vi "Laser.vi"() -> ()   [LabVIEW 2013]
doc: "Пограмма управления мишенью лазерного источника ионов."
uses:
  <vilib>/Utility/error.llb/DialogType.ctl
  <vilib>/Utility/inputDevices.llb/closeMouse.vi
  <vilib>/Utility/inputDevices.llb/mouseAcquire.vi
panel:
  in  "?":enum32{" Графики", " Настройки соединения"}(tab)
  out "Slide X axis":u8(slide) max=100 scale=0.0..100.0
  out "Slide Y axis":u8(slide) max=50 step=1
  in  "Коорд. y положение панели":u16
  in  "Коорд. X положение панели":u16
  in  "Add Button":bool
  in  "Коорд. Y":u16
  in  "Коорд. X":u16
  in  "размер, Y":dbl step=10.0
  in  "размер, X":dbl
  in  "Снимок":bool
  in  "Запись в файл":bool
  out "con err":bool caption="Connect"
  out "Con":bool
  out "warning1":string
  out "data out":string
  in  "thickness":u16 step=1
  out "Mouse on Pane pos Horizontal":i32
  out "Mouse on Pane pos Vertical":i32
  in  "in picture":picture
  in  "порт":u16=4001
  in  "IP-адрес":string="10.10.10.2"
  in  "Disconnect":bool caption="Disconn"
  out "Connected":bool
  in  "Connect":bool
  out "TCP error source":string
  in  "stop":bool
  out "read_error_indicator":bool
  in  "Connect 2":bool caption="Connect"
  in  "Компактный вид":bool
  out "resize Fl":bool caption="Disconn"
  in  "flag1":bool caption="Disconn"
  out "x+1":dbl
  out "connection ID":refnum<k5>
types:
  T1 = typedef "DialogType.ctl" = u16
  T2 = typedef "imagedata.ctl" = cluster{"image type":i32, "image depth":i32, "image":u8[], "mask":u8[], "colors":u32[], "Rectangle":cluster{"left":i16, "top":i16, "right":i16, "bottom":i16}}
  T3 = cluster{"Коорд. X положение панели":u16, "Коорд. y положение панели":u16}
  T4 = cluster{"Horizontal":i32, "Vertical":i32, "Scrolling":i32}
  T5 = typedef "LVRectTypeDef.ctl" = cluster{"Left":i16, "Top":i16, "Right":i16, "Bottom":i16}
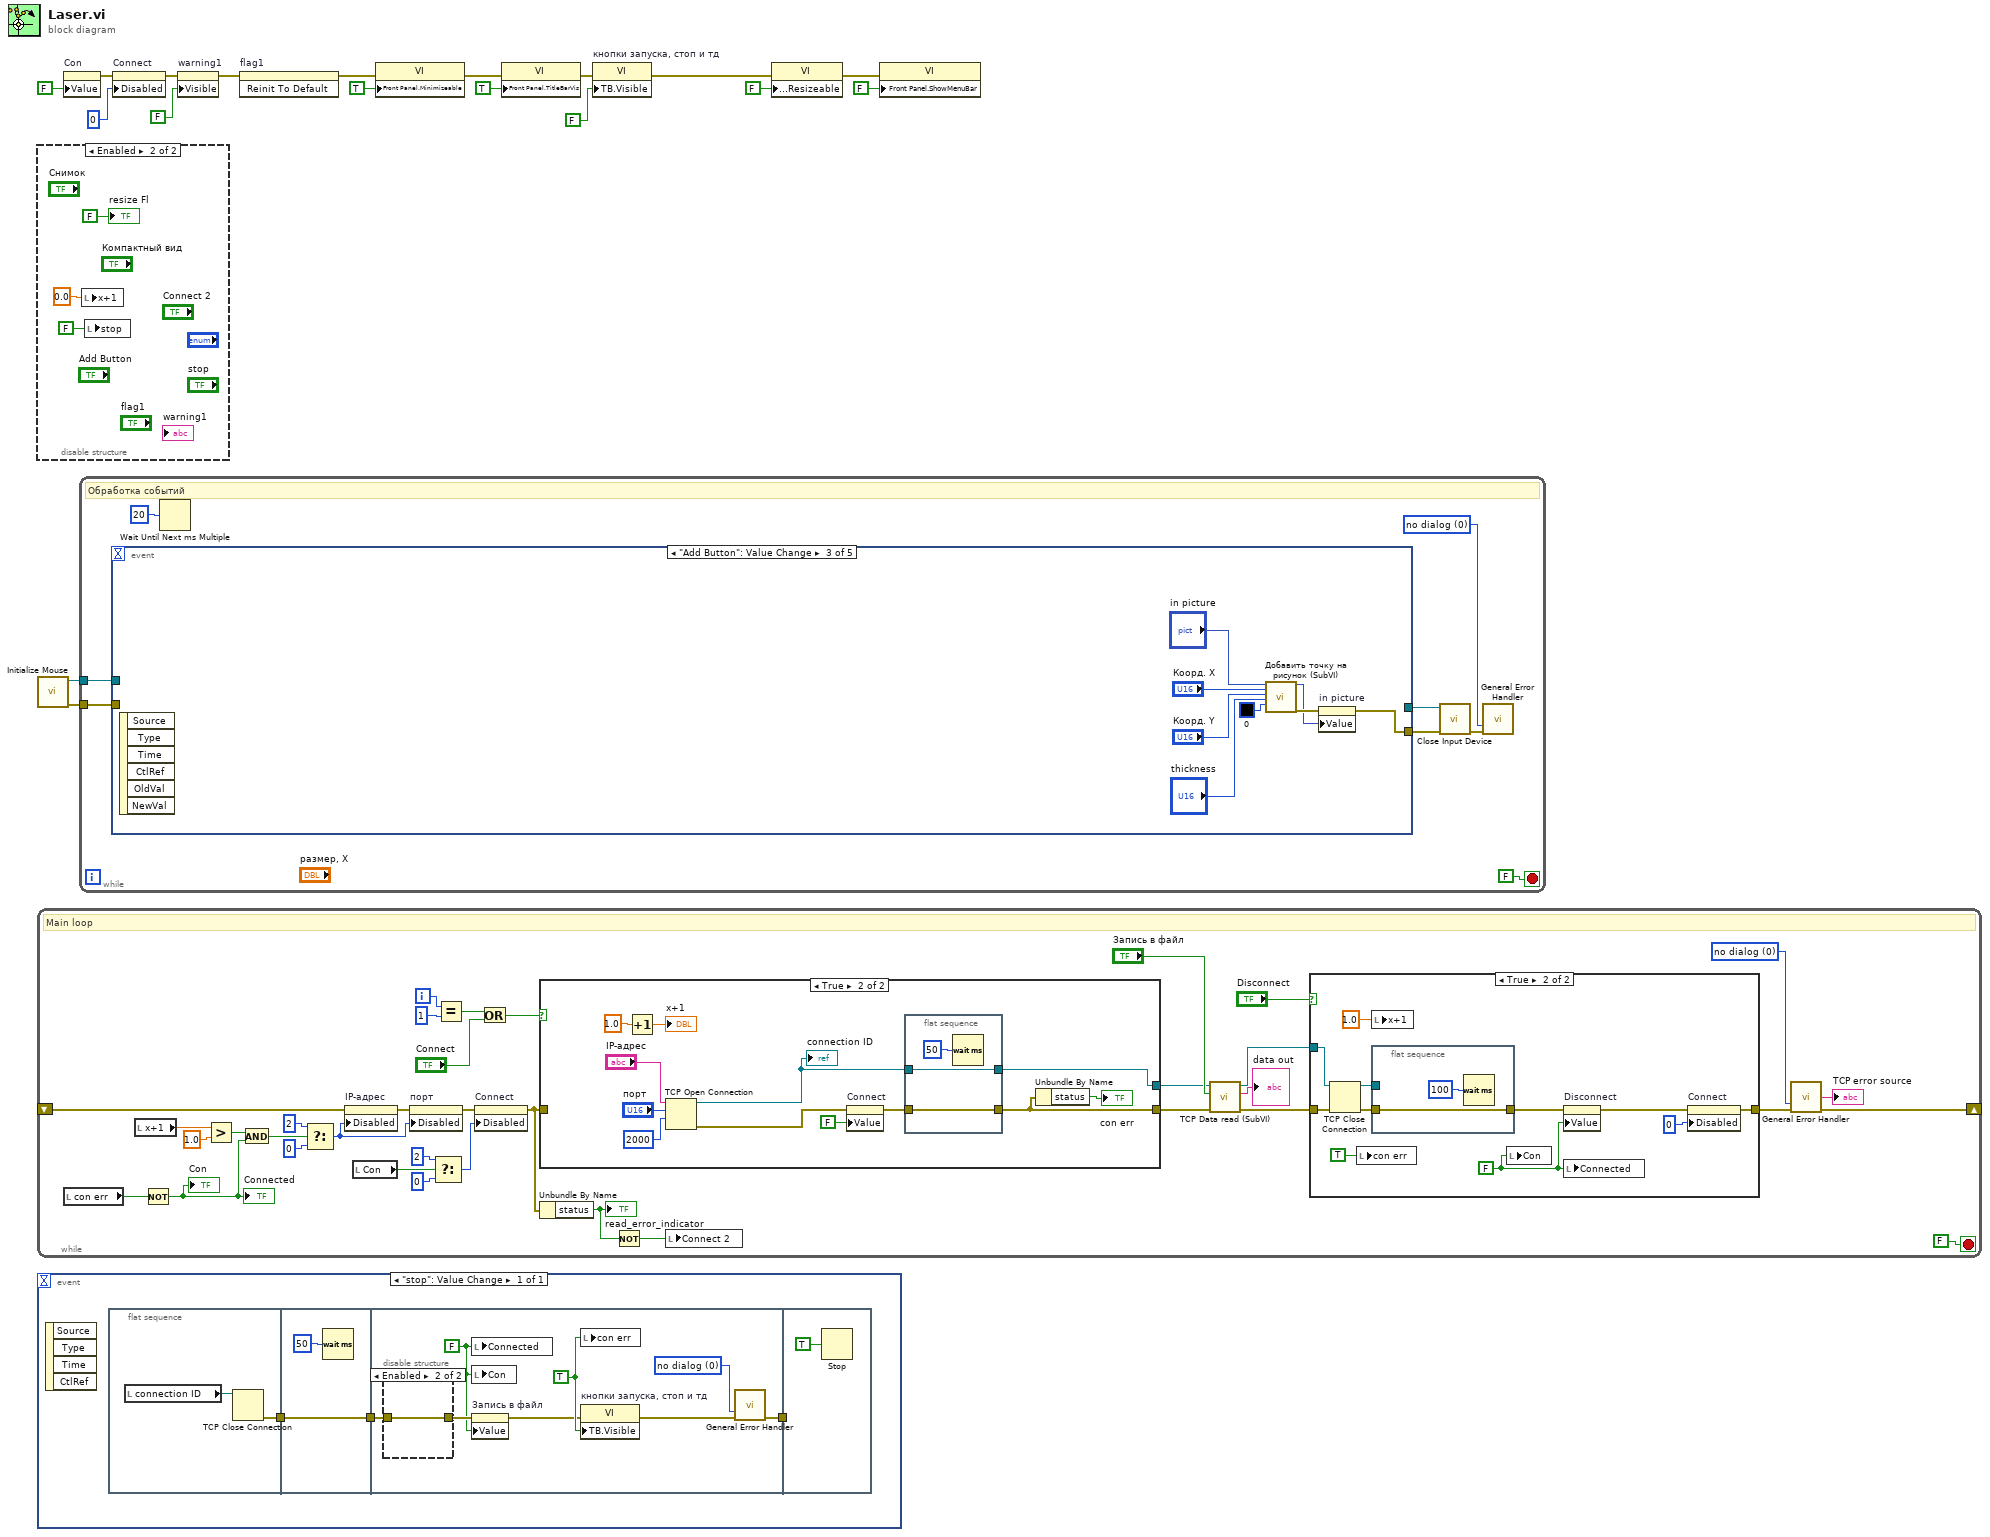
[diagram p0: block diagram]
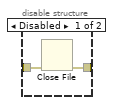
[diagram p3: hidden frame]
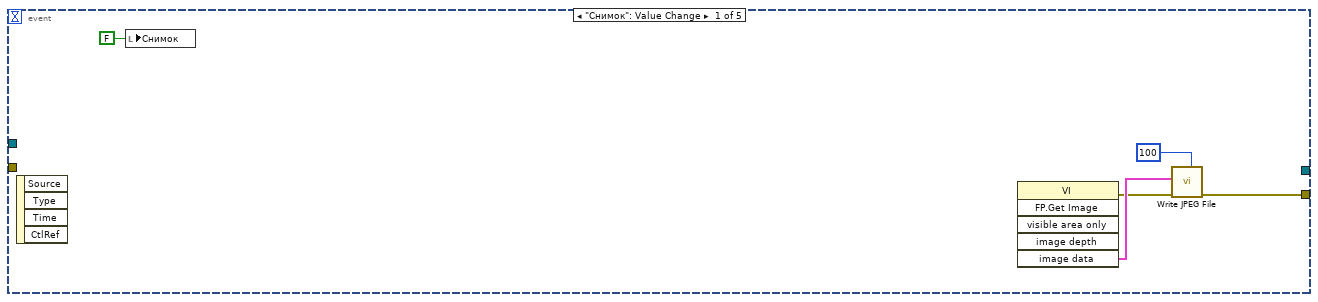
[diagram p4: hidden frame]
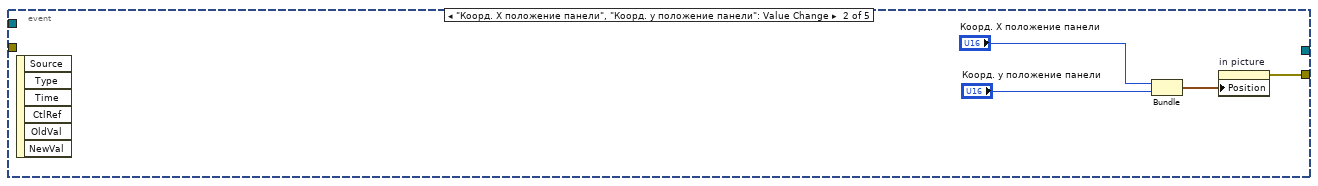
[diagram p5: hidden frame]
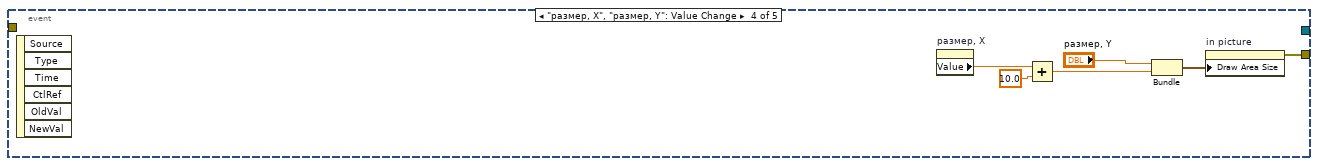
[diagram p6: hidden frame]
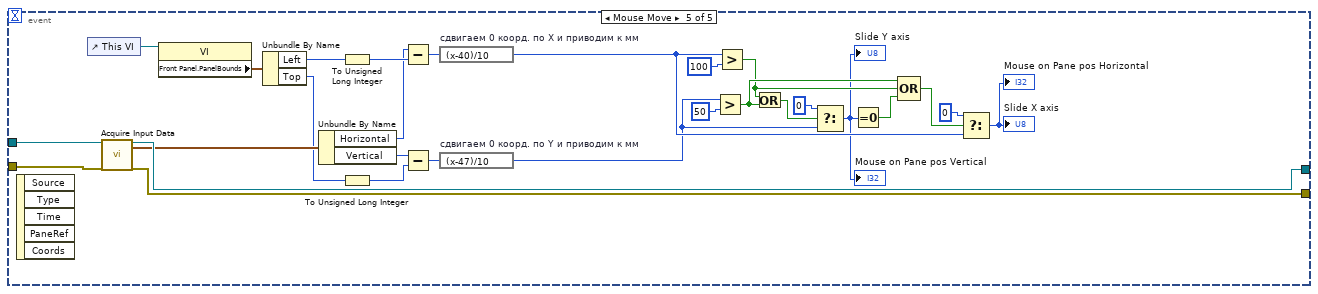
[diagram p7: hidden frame]
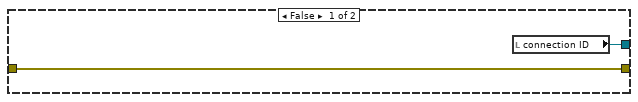
[diagram p8: hidden frame]
diagram:
  n1 = disable-structure shown="Enabled" {
    frame Disabled {
    }
    frame Enabled {
      n2 = local write "x+1"(0.0 ("x+1")) -> ()
      n3 = local write "stop"(FALSE ("Boolean")) -> ()
      "resize Fl" <- FALSE ("resize Fl")
    }
  }
  n4 = call <vilib>:"Initialize Mouse.vi"() -> ("error out"=w2:errorcluster, "device ID"=w1:refnum<k1>)  [unwired: 10 in]
  n5 = while {
    shift-right: [w32] -> _
    shift-left: _ -> [w30]
    i -> [w37]
    stop <- FALSE stop-if-true
    w33 = T1 0 items=["no dialog", "OK message", "continue or stop message", "OK message + warnings", "continue/stop + warnings"] ("type of dialog (OK msg:1)")
    # "Main loop"
    n6 = local read "con err"() -> (w54:bool)
    n7 = local read "x+1"() -> (w57:dbl)
    n8 = Not(x=w54) -> (.not. x?=w53:bool)
    "Connected" <- w53
    "Con" <- w53
    n9 = Greater?(x=w57, y=1.0) -> (0:w55:bool)
    n10 = And(x=w55, y=w53) -> (x .and. y?=w44:bool)
    n11 = Select(t=u8 2 ("Disabled"), s=w44, f=u8 0 ("Disabled")) -> (s? t:f=w43:u8)
    n12 = property on="IP-адрес" class="Str"(error in=w30, "Disabled"=w43) -> (error out=w42:errorcluster)  [unwired: 1 in, 1 out]
    n13 = local read "Con"() -> (w50:bool)
    n14 = property on="порт" class="DigNum (strict)"(error in=w42, "Disabled"=w43) -> (error out=w41:errorcluster)  [unwired: 1 in, 1 out]
    n15 = Select(t=u8 2 ("Disabled"), s=w50, f=u8 0 ("Disabled")) -> (s? t:f=w47:u8)
    n16 = Equal?(x=w37, y=1) -> (x = y?=w38:bool)
    n17 = property on="Connect" class="Bool (strict)"(error in=w41, "Disabled"=w47) -> (error out=w35:errorcluster)  [unwired: 1 in, 1 out]
    n18 = Or(x=w38, y="Connect") -> (x .or. y?=w40:bool)
    n19 = case shown="True" w40 {
      tunnel: [w59 w60] -> w28
      tunnel: [w58 w62] -> w25
      tunnel: w35 -> [w59 _]
      frame False {
        n20 = local read "connection ID"() -> (w58:refnum<k5>)
      }
      frame True {
        n21 = Increment(x=1.0) -> (x+1=→"x+1":dbl)
        n22 = TCP Open Connection(address="IP-адрес", remote port or service name="порт", timeout ms (60000)=2000) -> (connection ID=w63:refnum<k5>, error out=w65:errorcluster)  [unwired: 1 in, 1 out]
        "connection ID" <- w63
        n23 = property on="Connect" class="Bool (strict)"(error in=w65, "Value"=FALSE ("Connect")) -> (error out=w64:errorcluster)  [unwired: 1 in, 1 out]
        n24 = flat-sequence {
          tunnel: w64 -> [w73]
          tunnel: [w73] -> w60
          tunnel: w63 -> [w72]
          tunnel: [w72] -> w62
          frame #0 {
            n25 = Wait (ms)(milliseconds to wait=u32 50) -> ()  [unwired: 1 out]
          }
        }
        n26 = Unbundle By Name(w60) -> ("status"=→"con err":bool)
      }
    }
    n27 = Unbundle By Name(w35) -> ("status"=w29:bool)
    "read_error_indicator" <- w29
    n28 = Not(x=w29) -> (.not. x?=w52:bool)
    n29 = local write "Connect 2"(w52) -> ()
    n30 = call "TCP Data read (SubVI).vi"("error in (no error)"=w28, "Запись в файл"="Запись в файл", "TCP Network Connection in"=w25) -> ("error out"=w27:errorcluster, "Read data"=→"data out":string, "TCP Network Connection out"=w24:refnum<k5>)  [unwired: 5 in, 1 out]
    n31 = case shown="True" "Disconnect" {
      tunnel: [_ w77] -> w31
      tunnel: w27 -> [_ w76]
      tunnel: w24 -> [_ w75]
      frame False {
      }
      frame True {
        w78 = FALSE ("Disconnect")
        n32 = TCP Close Connection(connection ID=w75, error in (no error)=w76) -> (connection ID out=w81:refnum<k5>, error out=w80:errorcluster)  [unwired: 1 out]
        n33 = local write "con err"(TRUE ("con err")) -> ()
        n34 = local write "x+1"(1.0 ("1")) -> ()
        n35 = flat-sequence {
          tunnel: w81 -> [_]
          tunnel: w80 -> [w86]
          tunnel: [w86] -> w79
          frame #0 {
            n36 = Wait (ms)(milliseconds to wait=u32 100) -> ()  [unwired: 1 out]
          }
        }
        n37 = local write "Con"(w78) -> ()
        n38 = property on="Disconnect" class="Bool (strict)"(error in=w79, "Value"=w78) -> (error out=w82:errorcluster)  [unwired: 1 in, 1 out]
        n39 = local write "Connected"(w78) -> ()
        n40 = property on="Connect" class="Bool (strict)"(error in=w82, "Disabled"=u8 0) -> (error out=w77:errorcluster)  [unwired: 1 in, 1 out]
      }
    }
    n41 = call <vilib>:"General Error Handler.vi"("type of dialog (OK msg:1)"=w33, "error in (no error)"=w31) -> ("source out"=→"TCP error source":string, "error out"=w32:errorcluster)  [unwired: 12 out]
  }
  n42 = event shown="[0] \"stop\": Value Change" {
    selector: _ -> [_]
    dyn-events: _ -> [_]
    timeout: _ -> [_]
    event "stop": Value Change {
      n43 = event-data() -> ()  [unwired: 5 out]
      n44 = flat-sequence {
        tunnel: [w91] -> w90
        tunnel: w90 -> [w94]
        tunnel: [w94] -> w89
        tunnel: w89 -> [w97]
        tunnel: [w95] -> w88
        tunnel: w88 -> [_]
        frame #0 {
          n45 = local read "connection ID"() -> (w92:refnum<k5>)
          n46 = TCP Close Connection(connection ID=w92) -> (error out=w91:errorcluster)  [unwired: 1 in, 2 out]
        }
        frame #1 {
          n47 = Wait (ms)(milliseconds to wait=u32 50) -> ()  [unwired: 1 out]
        }
        frame #2 {
          w98 = T1 0 items=["no dialog", "OK message", "continue or stop message", "OK message + warnings", "continue/stop + warnings"] ("type of dialog (OK msg:1)")
          w101 = FALSE ("Запись в файл")
          w100 = TRUE ("Tool Bar:Visible")
          n48 = disable-structure shown="Enabled" {
            disable-tunnel: [w104 w105] -> w102
            disable-tunnel: w97 -> [w103 w105]
            frame Disabled {
              n49 = Close File(error in=w103) -> (error out=w104:errorcluster)  [unwired: 1 in, 1 out]
            }
            frame Enabled {
            }
          }
          n50 = local write "Connected"(w101) -> ()
          n51 = local write "Con"(w101) -> ()
          n52 = property on="Запись в файл" class="Bool (strict)"(error in=w102, "Value"=w101) -> (error out=w99:errorcluster)  [unwired: 1 in, 1 out]
          n53 = local write "con err"(w100) -> ()
          n54 = property on="кнопки запуска, стоп и тд" class="VI"(error in=w99, "TB.Visible"=w100) -> (error out=w96:errorcluster)  [unwired: 1 in, 1 out]
          n55 = call <vilib>:"General Error Handler.vi"("type of dialog (OK msg:1)"=w98, "error in (no error)"=w96) -> ("error out"=w95:errorcluster)  [unwired: 13 out]
        }
        frame #3 {
          n56 = Stop(stop? (T)=TRUE) -> ()
        }
      }
    }
  }
  n57 = property on="Con" class="Bool (strict)"("Value"=FALSE ("Connected")) -> (error out=w5:errorcluster)  [unwired: 2 in, 1 out]
  n58 = while {
    tunnel: w2 -> [w111]
    tunnel: w1 -> [w110]
    stop <- FALSE stop-if-true
    w112 = T1 0 items=["no dialog", "OK message", "continue or stop message", "OK message + warnings", "continue/stop + warnings"] ("type of dialog (OK msg:1)")
    # "Обработка событий"
    n59 = event shown="[2] \"Add Button\": Value Change" {
      selector: _ -> [_ _ _ _ _]
      dyn-events: _ -> [_ _ _ _ _]
      timeout: _ -> [_ _ _ _ _]
      tunnel: [w115 w122 w124 w137 w157] -> w109
      tunnel: w111 -> [_ _ _ _ w164]
      tunnel: w110 -> [_ _ _ _ w165]
      tunnel: [_ _ _ _ w163] -> w107
      event "Снимок": Value Change {
        n60 = event-data() -> ()  [unwired: 5 out]
        n61 = local write "Снимок"(FALSE ("Снимок")) -> ()
        n62 = invoke class="VI" method="FP.Get Image"() -> (error out=w116:errorcluster, "image data"=w117:T2)  [unwired: 6 in, 4 out]
        n63 = call <vilib>:"Write JPEG File.vi"("quality (80)"=100, "error in (no error)"=w116, "image data"=w117) -> ("error out"=w115:errorcluster)  [unwired: 1 in, 7 out]
      }
      event "Коорд. X положение панели", "Коорд. y положение панели": Value Change {
        n64 = event-data() -> ()  [unwired: 7 out]
        n65 = Bundle("Коорд. X положение панели"="Коорд. X положение панели", "Коорд. y положение панели"="Коорд. y положение панели") -> (w123:T3)  [unwired: 1 in]
        n66 = property on="in picture" class="Pict"("Position"=w123) -> (error out=w122:errorcluster)  [unwired: 2 in, 1 out]
      }
      event "Add Button": Value Change {
        n67 = event-data() -> ()  [unwired: 7 out]
        n68 = call "Добавить точку на рисунок (SubVI).vi"("in picture"="in picture", "dot х"="Коорд. X", "dot y"="Коорд. Y", "thickness"="thickness", "цвет"=u32 0) -> ("out picture"=w130:picture, "error out"=w131:errorcluster)  [unwired: 13 in]
        n69 = property on="in picture" class="Pict"(error in=w131, "Value"=w130) -> (error out=w124:errorcluster)  [unwired: 1 in, 1 out]
      }
      event "размер, X", "размер, Y": Value Change {
        n70 = event-data() -> ()  [unwired: 7 out]
        n71 = property on="размер, X" class="DigNum (strict)"() -> ("Value"=w135:dbl)  [unwired: 2 in, 2 out]
        n72 = Add(x=w135, y=10.0) -> (x+y=w133:dbl)
        n73 = Bundle("размер, Y"="размер, Y", w133) -> (w134:cluster{"размер, Y":dbl, dbl})  [unwired: 1 in]
        n74 = property on="in picture" class="Pict"("Draw Area Size"=w134) -> (error out=w137:errorcluster)  [unwired: 2 in, 1 out]
      }
      event Mouse Move {
        n75 = event-data() -> ()  [unwired: 6 out]
        n76 = control-ref of="This VI"() -> (w161:refnum<vi>)
        n77 = call-poly <vilib>:"Acquire Input Data.vi"("device ID"=w165, "error in (no error)"=w164) -> ("device ID"=w163:refnum<k1>, "axis info"=w162:T4, "error out"=w157:errorcluster)  [unwired: 14 in, 1 out]
        n78 = property class="VI"(reference=w161) -> ("Front Panel.PanelBounds"=w160:T5)  [unwired: 1 in, 2 out]
        n79 = Unbundle By Name(w160) -> ("Left"=w159:i16, "Top"=w158:i16)
        n80 = Unbundle By Name(w162) -> ("Horizontal"=w155:i32, "Vertical"=w153:i32)
        n81 = To Unsigned Long Integer(number=w159) -> (unsigned 32bit integer=w156:u32)
        n82 = To Unsigned Long Integer(number=w158) -> (unsigned 32bit integer=w154:u32)
        n83 = Subtract(x=w155, y=w156) -> (x-y=w152:u32)
        n84 = Subtract(x=w153, y=w154) -> (x-y=w151:u32)
        n85 = expression code="(x-40)/10" "сдвигаем 0 коорд. по X и приводим к мм"(w152) -> (w146:u32)
        n86 = expression code="(x-47)/10" "сдвигаем 0 коорд. по Y и приводим к мм"(w151) -> (w145:u32)
        n87 = Greater?(x=w145, y=50) -> (0:w143:bool)
        n88 = Greater?(x=w146, y=100) -> (0:w142:bool)
        n89 = Or(x=w142, y=w143) -> (x .or. y?=w144:bool)
        n90 = Select(t=0, s=w144, f=w145) -> (s? t:f=w139:u32)
        "Mouse on Pane pos Vertical" <- w139
        "Slide Y axis" <- w139
        n91 = Equal To 0?(x=w139) -> (x = 0?=w141:bool)
        n92 = Compound Arithmetic op=OR(w143, w142, w141) -> (w140:bool)
        n93 = Select(t=0, s=w140, f=w146) -> (s? t:f=→"Mouse on Pane pos Horizontal" →"Slide X axis":u32)
      }
    }
    n94 = Wait Until Next ms Multiple(millisecond multiple=u32 20) -> ()  [unwired: 1 out]
    n95 = call-poly <vilib>:"Close Input Device.vi"("error in (no error)"=w109, "device ID"=w107) -> ("error out"=w108:errorcluster)  [unwired: 8 in]
    n96 = call <vilib>:"General Error Handler.vi"("type of dialog (OK msg:1)"=w112, "error in (no error)"=w108) -> ()  [unwired: 9 in, 5 out]
  }
  n97 = property on="Connect" class="Bool (strict)"(error in=w5, "Disabled"=u8 0) -> (error out=w10:errorcluster)  [unwired: 1 in, 1 out]
  n98 = property on="warning1" class="Str"(error in=w10, "Visible"=FALSE) -> (error out=w3:errorcluster)  [unwired: 1 in, 1 out]
  n99 = invoke on="flag1" class="Bool (strict)" method="Reinit To Default"(error in=w3) -> (error out=w4:errorcluster)  [unwired: 2 in, 2 out]
  n100 = property class="VI"(error in=w4, "Front Panel.Minimizeable"=TRUE ("Front Panel Window:Minimizable")) -> (error out=w9:errorcluster)  [unwired: 1 in, 1 out]
  n101 = property class="VI"(error in=w9, "Front Panel.TitleBarVis"=TRUE ("Front Panel Window:Title Bar Visible")) -> (error out=w8:errorcluster)  [unwired: 1 in, 1 out]
  n102 = property on="кнопки запуска, стоп и тд" class="VI"(error in=w8, "TB.Visible"=FALSE ("Tool Bar:Visible")) -> (error out=w7:errorcluster)  [unwired: 1 in, 1 out]
  n103 = property class="VI"(error in=w7, "Front Panel.Resizeable"=FALSE ("Front Panel Window:Resizable")) -> (error out=w6:errorcluster)  [unwired: 1 in, 1 out]
  n104 = property class="VI"(error in=w6, "Front Panel.ShowMenuBar"=FALSE ("Front Panel Window:Show Menu Bar")) -> ()  [unwired: 1 in, 2 out]
